vi "DeleteAll.vi"(8 "error in (no error)":errorcluster, 11 "ResultTree in":refnum<class "ResultTree.lvclass">) -> (0 "error out":errorcluster, 3 "ResultTree out":refnum<class "ResultTree.lvclass">)   [LabVIEW 2019, in "ResultTree.lvclass"]
doc: "Deletes all items in the tree."
uses:
  ResultTree.lvclass
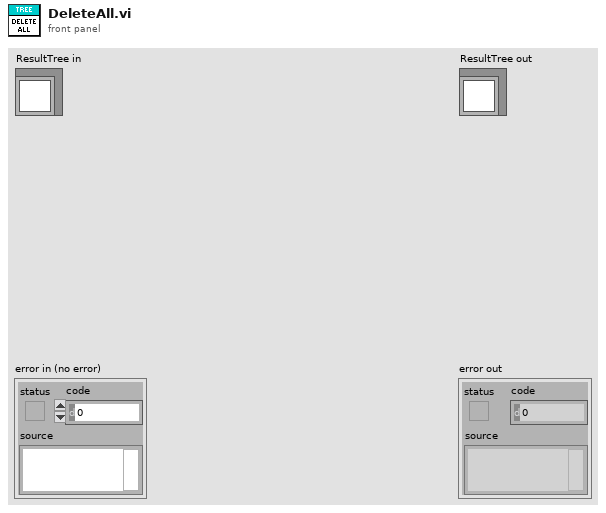
[diagram p1: front panel]
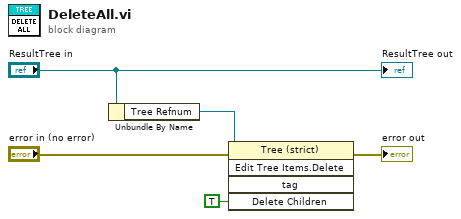
[diagram p0: block diagram]
diagram:
  n1 = Unbundle By Name("ResultTree in") -> ("Tree Refnum"=w1:refnum<vi>)
  n2 = invoke class="Tree (strict)" method="Edit Tree Items.Delete"(reference=w1, error in="error in (no error)", "Delete Children"=TRUE ("Delete Children?")) -> (error out=→"error out":errorcluster)  [unwired: 2 in, 4 out]
  "ResultTree out" <- "ResultTree in"
